vi "Inspect Address Pads.vi"(7 "Console Log in":refnum<class "Console Log.lvclass">, 8 "error in":errorcluster, 10 "Module Data In":T6, 11 "Potting Procedure in":refnum<class "Potting Procedure.lvclass">) -> (0 "error out":errorcluster, 2 "Module Data Out":T6, 3 "Potting Procedure out":refnum<class "Potting Procedure.lvclass">, 5 "Console Log out":refnum<class "Console Log.lvclass">)   [LabVIEW 2011, in "Potting Procedure.lvclass"]
uses:
  Potting Procedure.lvclass
  Shared Components/Utils/Type Definitions/Multi-Fiducial Image.ctl
  Shared Components/Utils/Type Definitions/Physical Image.ctl
  Shared Components/Vec3d Class/Vec3d Class.lvclass
  <vilib>/vision/Image Controls.llb/IMAQ Image.ctl
  Shared Components/Utils/Type Definitions/Fiducial with Source.ctl
  Shared Components/Utils/Type Definitions/Fiducial Image.ctl
  UI Classes/Console Log/Console Log.lvclass
  Shared Components/Gantry Class/Gantry Class.lvclass
  Shared Components/WorkTable Class/WorkTable Class.lvclass
  Shared Components/CameraTool Class/Take Area Image.vi
  Shared Components/CameraTool Class/CameraTool Class.lvclass
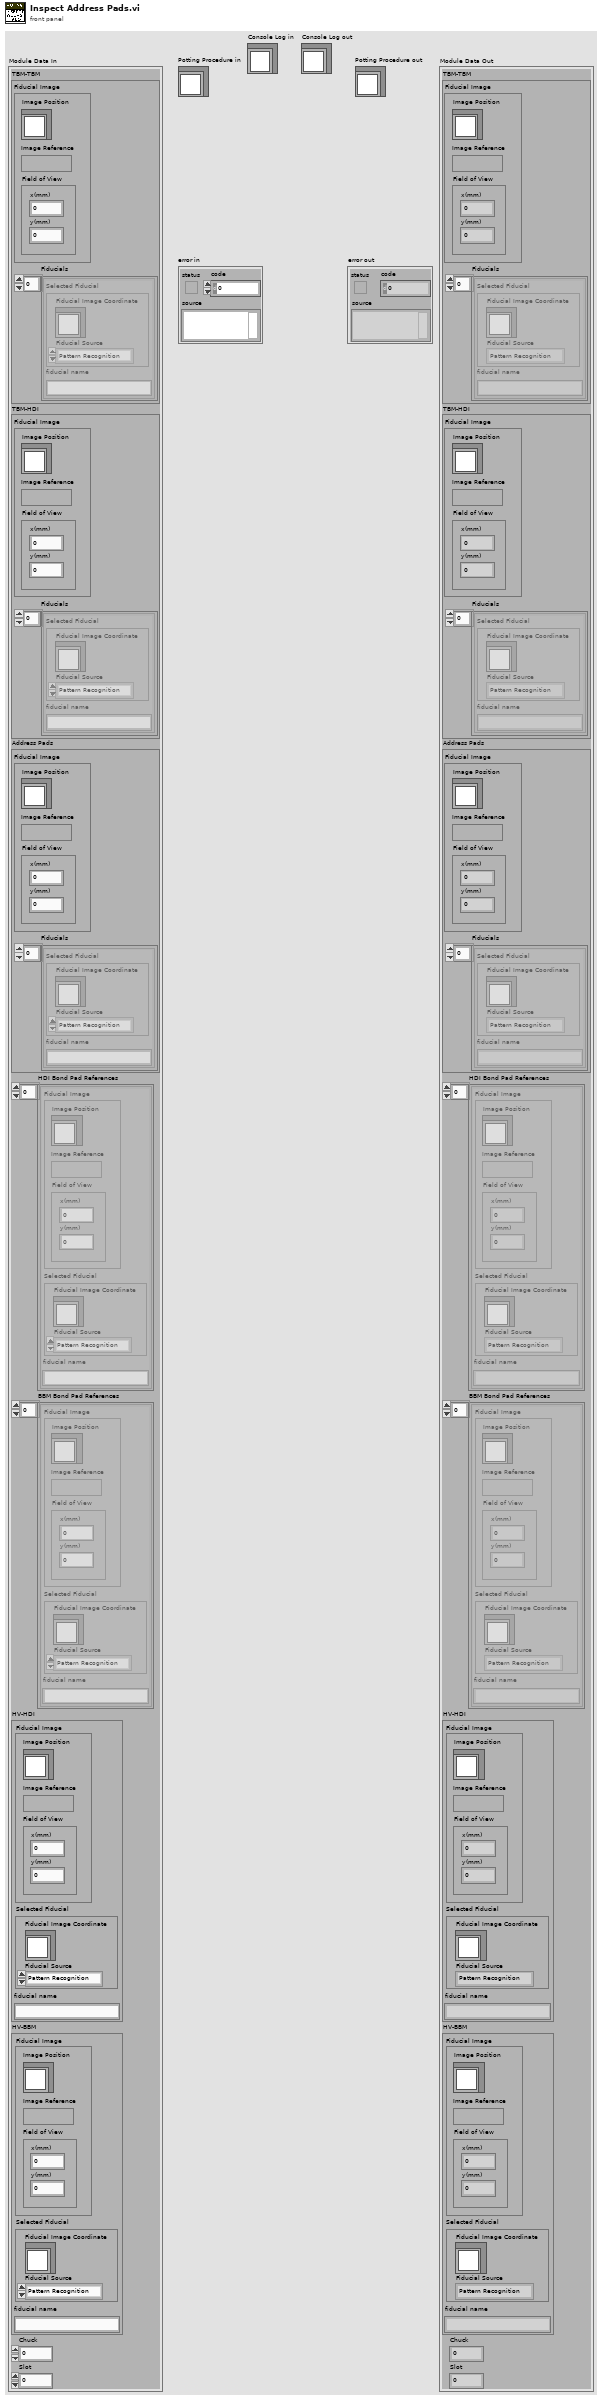
[diagram p1: front panel]
types:
  T1 = typedef "Multi-Fiducial Image.ctl" = cluster{"Fiducial Image":T2, "Fiducials":cluster{"Selected Fiducial":T4, "fiducial name":string}[]}
  T2 = typedef "Physical Image.ctl" = cluster{"Image Position":refnum<class "Vec3d Class.lvclass">, "Image Reference":T3, "Field of View":cluster{"x(mm)":dbl, "y(mm)":dbl}}
  T3 = typedef "IMAQ Image.ctl" = refnum<image>
  T4 = typedef "Fiducial with Source.ctl" = cluster{"Fiducial Image Coordinate":refnum<class "Vec3d Class.lvclass">, "Fiducial Source":enum16{"Pattern Recognition", "User", "Error", "Default"}}
  T5 = typedef "Fiducial Image.ctl" = cluster{"Fiducial Image":T2, "Selected Fiducial":T4, "fiducial name":string}
  T6 = cluster{"TBM-TBM":T1, "TBM-HDI":T1, "Address Pads":T1, "HDI Bond Pad References":T5[], "BBM Bond Pad References":T5[], "HV-HDI":T5, "HV-BBM":T5, "Chuck":i32, "Slot":i32}
  T7 = enum16{"Pattern Recognition", "User", "Error", "Default"}
  T8 = cluster{"Selected Fiducial":T4, "fiducial name":string}
  T9 = typedef "Worktable_Module Slot.ctl" = cluster{"Slot State":enum16{"Empty", "Unglued", "Stamped", "PartOnTop", "Weighted", "Unpotted", "Potted"}, "BBM Type":enum16{"None", "BBM", "GlassSlide"}, "HDI Type":enum16{"None", "HDI", "Polyimide"}, "Vacuum Channel":u8, "Location/Orientation BBM":T10, "Location/Orientation HDI":T10, "S/N":string}
  T10 = typedef "Position_Orientation.ctl" = cluster{"Center":refnum<class "Vec3d Class.lvclass">, "Orientation":refnum<class "Orient3d Class.lvclass">}
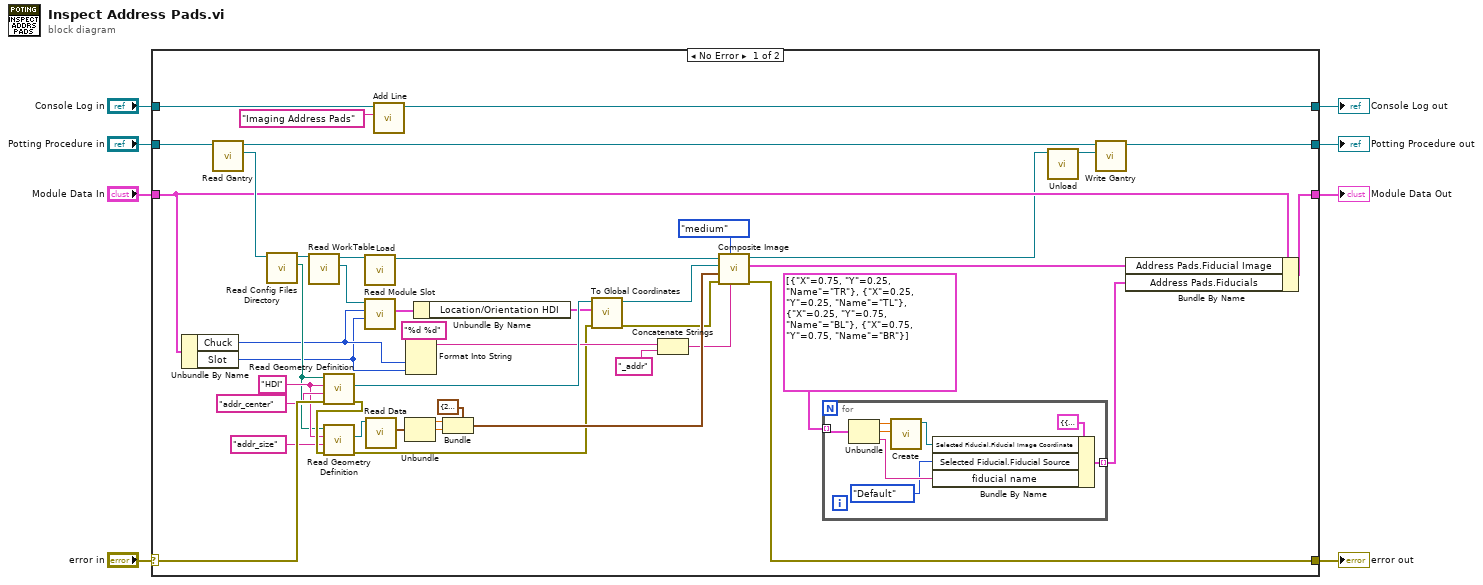
[diagram p0: block diagram]
diagram:
  n1 = case shown="No Error" "error in" {
    selector: "error in" -> [w48 w64]
    tunnel: [w13 w64] -> w6
    tunnel: [w19 w63] -> w8
    tunnel: "Potting Procedure in" -> [w52 w63]
    tunnel: "Module Data In" -> [w23 w62]
    tunnel: [w20 w62] -> w7
    tunnel: "Console Log in" -> [w11 w61]
    tunnel: [w10 w61] -> w1
    frame No Error {
      w44 = "HDI" ("Part")
      n2 = Unbundle By Name(w23) -> ("Chuck"=w25:i32, "Slot"=w24:i32)
      n3 = call-dynamic "Read Gantry.vi"("Potting Procedure in"=w52) -> ("Gantry"=w49:refnum<class "Gantry Class.lvclass">, "Potting Procedure out"=w18:refnum<class "Potting Procedure.lvclass">)  [unwired: 8 in, 1 out]
      n4 = call-dynamic "Read Config Files Directory.vi"("Gantry Class in"=w49) -> ("Config Files Directory"=w43:path, "Gantry Class out"=w36:refnum<class "Gantry Class.lvclass">)  [unwired: 8 in, 1 out]
      n5 = call-dynamic "Read WorkTable.vi"("Gantry Class in"=w36) -> ("WorkTable Class.lvclass"=w34:refnum<class "WorkTable Class.lvclass">, "Gantry Class out"=w35:refnum<class "Gantry Class.lvclass">)  [unwired: 8 in, 1 out]
      n6 = call "Read Geometry Definition.vi"("error in"=w48, "Feature"="addr_center", "Part"=w44, "Config Location"=w43) -> ("error out"=w47:errorcluster, "Feature Coordinates"=w32:refnum<class "Vec3d Class.lvclass">)  [unwired: 6 in]
      n7 = call "Read Geometry Definition.vi"("error in"=w47, "Feature"="addr_size", "Part"=w44, "Config Location"=w43) -> ("error out"=w16:errorcluster, "Feature Coordinates"=w42:refnum<class "Vec3d Class.lvclass">)  [unwired: 6 in]
      n8 = call "Load.vi"("Gantry In"=w35) -> ("CameraTool out"=w51:refnum<class "CameraTool Class.lvclass">)  [unwired: 9 in, 1 out]
      n9 = call-dynamic "Read Module Slot.vi"("slot"=w24, "chuck"=w25, "WorkTable in"=w34) -> ("Module Slot"=w33:T9)  [unwired: 6 in, 2 out]
      n10 = call-dynamic "Read Data.vi"("Vec3d Class in"=w42) -> ("Data"=w41:cluster{"X":dbl, "Y":dbl, "Z":dbl})  [unwired: 8 in, 2 out]
      n11 = call "Add Line.vi"("String"="Imaging Address Pads", "Console Log in"=w11) -> ("Console Log out"=w10:refnum<class "Console Log.lvclass">)  [unwired: 8 in, 1 out]
      n12 = Unbundle(w41) -> ("X"=w40:dbl, "Y"=w39:dbl)  [unwired: 1 out]
      n13 = Format Into String(format string="%d %d", w25, w24) -> (resulting string=w27:string)  [unwired: 2 in, 1 out]
      n14 = Unbundle By Name(w33) -> ("Location/Orientation HDI"=w31:T10)
      n15 = Bundle(cluster=cluster{"Size-X(mm)":dbl, "Size-Y(mm)":dbl} {"Size-X(mm)"=20.0, "Size-Y(mm)"=20.0} ("Field of View"), "Size-X(mm)"=w40, "Size-Y(mm)"=w39) -> (w38:cluster{"Size-X(mm)":dbl, "Size-Y(mm)":dbl})
      n16 = call "To Global Coordinates.vi"("error in"=w16, "Center/Orientation"=w31, "Local Coordinates"=w32) -> ("error out"=w30:errorcluster, "Global Coordinates"=w14:refnum<class "Vec3d Class.lvclass">)  [unwired: 7 in]
      n17 = Concatenate Strings(w27, "_addr" ("string")) -> (w26:string)
      n18 = call-poly "Composite Image.vi"("Image Name"=w26, "Quality"=enum16{"perfect", "medium", "low"}."medium", "error in"=w30, "Field of View"=w38, "Image Center"=w14, "CameraTool in"=w51) -> ("error out"=w13:errorcluster, "Physical Image"=w22:T2, "CameraTool out"=w15:refnum<class "CameraTool Class.lvclass">)  [unwired: 3 in]
      n19 = for {
        tunnel: cluster{"X":dbl, "Y":dbl, "Name":string}[] [{"X"=0.75, "Y"=0.25, "Name"="TR"}, {"X"=0.25, "Y"=0.25, "Name"="TL"}, {"X"=0.25, "Y"=0.75, "Name"="BL"}, {"X"=0.75, "Y"=0.75, "Name"="BR"}] -> [w59] mode=indexing
        tunnel: [w53] -> w12 mode=indexing
        n20 = Unbundle(w59) -> ("X"=w57:dbl, "Y"=w58:dbl, "Name"=w55:string)
        n21 = call "Create.vi"("Y"=w58, "X"=w57) -> ("Vec3d Class out"=w56:refnum<class "Vec3d Class.lvclass">)  [unwired: 8 in, 1 out]
        n22 = Bundle By Name(cluster=T8 {"Selected Fiducial"={"Fiducial Image Coordinate"=refnum, "Fiducial Source"=enum."Pattern Recognition"}, "fiducial name"=""} ("Fiducial"), "Selected Fiducial.Fiducial Image Coordinate"=w56, "Selected Fiducial.Fiducial Source"=T7."Default", "fiducial name"=w55) -> (w53:T8)
      }
      n23 = call "Unload.vi"("CameraTool in"=w15) -> ("Gantry out"=w17:refnum<class "Gantry Class.lvclass">)  [unwired: 9 in, 1 out]
      n24 = call-dynamic "Write Gantry.vi"("Gantry"=w17, "Potting Procedure in"=w18) -> ("Potting Procedure out"=w19:refnum<class "Potting Procedure.lvclass">)  [unwired: 8 in, 1 out]
      n25 = Bundle By Name(cluster=w23, "Address Pads.Fiducial Image"=w22, "Address Pads.Fiducials"=w12) -> (w20:T6)
    }
    frame Error {
    }
  }
  "error out" <- w6
  "Potting Procedure out" <- w8
  "Module Data Out" <- w7
  "Console Log out" <- w1
